vi "query_vectorsearch.vi"(0 "vector_qdrant in":refnum<class "vector_qdrant.lvclass">, 5 "collection_name":string, 7 "vector":dbl[](array[numeric]), 9 "limit":u32, 11 "error in":errorcluster) -> (4 "vector_qdrant out":refnum<class "vector_qdrant.lvclass">, 6 "results":T1[](array[typedef]), 15 "error out":errorcluster)   [LabVIEW 2020, in "vector_qdrant.lvclass"]
uses:
  vector_qdrant.lvclass
  abstract_vector_base/search result.ctl
  abstract_vector_base/vector.ctl
  vector_qdrant.lvclass/vector_qdrant.ctl
  <vilib>/httpClient/POSTBuffer.vi
  <vilib>/httpClient/LabVIEWHTTPClient.lvlib
  abstract_vector_base/abstract_vector_base.lvclass
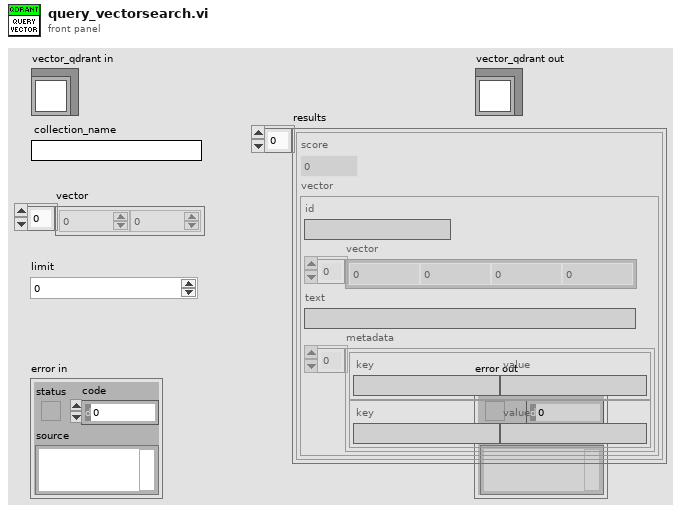
[diagram p1: front panel]
types:
  T1 = typedef "abstract_vector_base.lvclass/search result.ctl" = cluster{"score":dbl, "vector":T2}
  T2 = typedef "abstract_vector_base.lvclass/vector.ctl" = cluster{"id":string, "vector":dbl[], "text":string, "metadata":cluster{"key":string, "value":string}[]}
  T3 = typedef "LabVIEWHTTPClient.lvlib/ClientHandle.ctl" = refnum<k1>
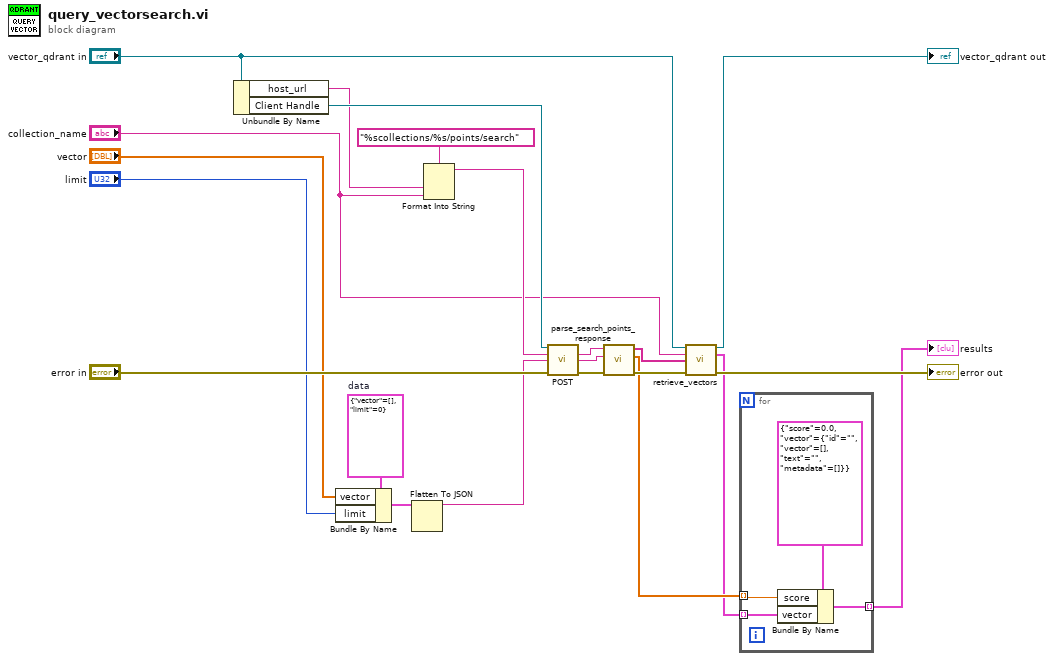
[diagram p0: block diagram]
diagram:
  w18 = cluster{"vector":dbl[], "limit":u32} {"vector"=[], "limit"=0}  # data
  n1 = Unbundle By Name("vector_qdrant in") -> ("host_url"=w19:string, "Client Handle"=w21:T3)
  n2 = Bundle By Name(cluster=w18, "vector"="vector", "limit"="limit") -> (w15:cluster{"vector":dbl[], "limit":u32})
  n3 = Flatten To JSON(anything=w15) -> (JSON string=w14:string)  [unwired: 2 in, 1 out]
  n4 = Format Into String(format string="%scollections/%s/points/search", w19, "collection_name") -> (resulting string=w13:string)  [unwired: 2 in, 1 out]
  n5 = call-poly <vilib>:"POST.vi"("client handle"=w21, "url"=w13, "buffer"=w14, "error in (no error)"="error in") -> ("headers"=w11:string, "body"=w10:string, "error out"=w12:errorcluster)  [unwired: 8 in, 1 out]
  n6 = call "parse_search_points_response.vi"("error in (no error)"=w12, "body"=w10, "headers"=w11) -> ("error out"=w7:errorcluster, "scores"=w3:dbl[], "ids"=w5:string[])  [unwired: 6 in]
  n7 = call-dynamic "retrieve_vectors.vi"("vector_qdrant in"="vector_qdrant in", "colection_name"="collection_name", "ids"=w5, "error in (no error)"=w7) -> ("vector_qdrant out"=→"vector_qdrant out":refnum<class "vector_qdrant.lvclass">, "Vectors"=w2:T2[], "error out"=→"error out":errorcluster)  [unwired: 9 in]
  n8 = for {
    tunnel: w3 -> [w25] mode=indexing
    tunnel: w2 -> [w24] mode=indexing
    tunnel: [w23] -> w1 mode=indexing
    n9 = Bundle By Name(cluster=T1 {"score"=0.0, "vector"={"id"="", "vector"=[], "text"="", "metadata"=[]}} ("response"), "score"=w25, "vector"=w24) -> (w23:T1)
  }
  "results" <- w1
